vi "Tags.vi"(8 "error in (no error)":errorcluster, 11 "Node Ptr":T1 format="%.0x") -> (0 "error out":errorcluster)   [LabVIEW 2019, in "OPC UA Client Addon System Explorer.lvlib"]
uses:
  OPC UA Client Addon System Explorer.lvlib
  <vilib>/NI VeriStand/Custom Device API/Custom Device API.lvlib
  <vilib>/NI VeriStand/Custom Device API/Custom Device Item Ref.ctl
panel:
  in  "SHDocVw.IWebBrowser":refnum<k7>(container)
types:
  T1 = typedef "Custom Device API.lvlib/Custom Device Item Ref.ctl" = u64
  T2 = typedef "Custom Device API.lvlib/Custom Device Commands.ctl" = enum16{"Default", "Item renamed", "Shutdown", "Dynamic button pressed"}
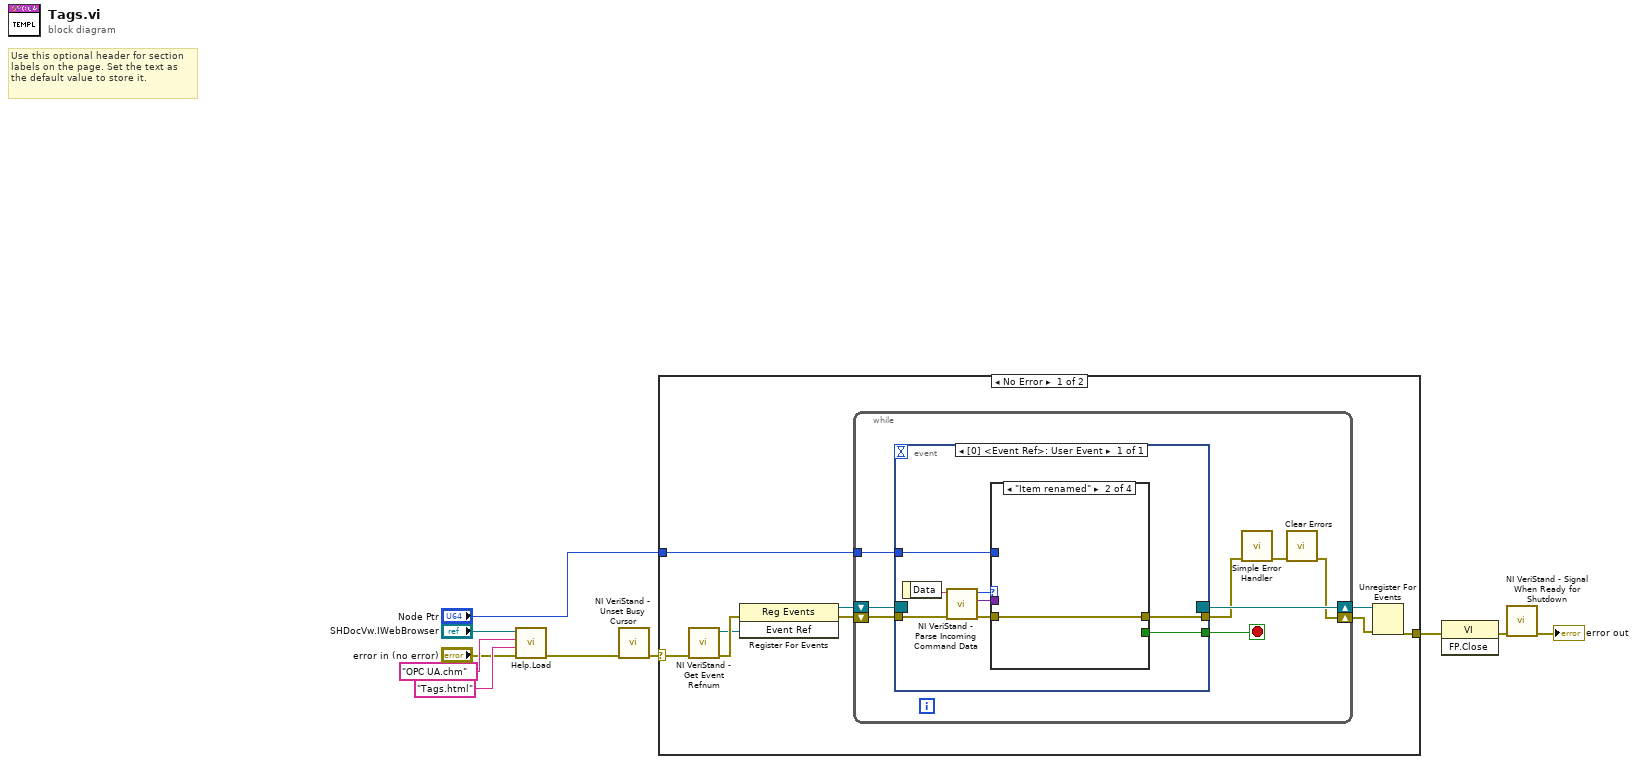
[diagram p0: block diagram]
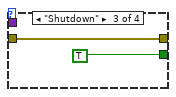
[diagram p3: hidden frame]
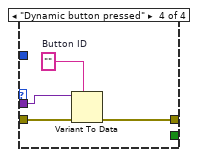
[diagram p4: hidden frame]
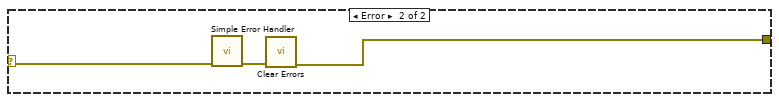
[diagram p5: hidden frame]
diagram:
  # "Use this optional header for section labels on the page. Set the text as the default value to store it."
  n1 = call "Help.Load.vi"("error in (no error)"="error in (no error)", "HTML File"="Tags.html" ("Main CHM File"), "Main CHM File"="OPC UA.chm", "SHDocVw.IWebBrowser2"="SHDocVw.IWebBrowser") -> ("error out"=w2:errorcluster)  [unwired: 7 in]
  n2 = call <vilib>:"NI VeriStand - Unset Busy Cursor.vi"("error in (no error)"=w2) -> ("error out"=w7:errorcluster)  [unwired: 10 out]
  n3 = case shown="No Error" w7 {
    selector: w7 -> [w11 w46]
    tunnel: [w16 w44] -> w10
    tunnel: "Node Ptr" -> [w12 _]
    frame No Error {
      n4 = call <vilib>:"NI VeriStand - Get Event Refnum.vi"("error in (no error)"=w11) -> ("error out"=w19:errorcluster, "Event Ref"=w15:refnum<user-event>)  [unwired: 9 out]
      n5 = register-events(error in=w19, w15) -> (reference out=w13:refnum<event-registration>, error out=w14:errorcluster)  [unwired: 1 in]
      n6 = while {
        tunnel: w12 -> [w23]
        shift-right: [w20] -> w17
        shift-left: w14 -> [w26]
        shift-right: [w27] -> w18
        shift-left: w13 -> [w25]
        stop <- w24 stop-if-true
        n7 = event shown="[0] <Event Ref>: User Event" {
          selector: w25 -> [_]
          dyn-events: [_] -> w27
          timeout: _ -> [_]
          tunnel: w26 -> [w35]
          tunnel: [w31] -> w24
          tunnel: [w30] -> w22
          tunnel: w23 -> [w29]
          event User Event {
            n8 = event-data() -> ("Data"=w34:string)  [unwired: 1 out]
            n9 = call <vilib>:"NI VeriStand - Parse Incoming Command Data.vi"("error in (no error)"=w35, "Incoming data"=w34) -> ("error out"=w33:errorcluster, "Outgoing data"=w28:variant, "Action"=w32:T2)  [unwired: 7 out]
            n10 = case shown="\"Item renamed\"" w32 {
              tunnel: w33 -> [w36 w37 w38 w43]
              tunnel: [_ _ TRUE _] -> w31
              tunnel: [w36 w37 w38 w40] -> w30
              tunnel: w29 -> [_ _ _ _]
              tunnel: w28 -> [_ _ _ w42]
              frame "Default", Default {
              }
              frame "Item renamed" {
              }
              frame "Shutdown" {
              }
              frame "Dynamic button pressed" {
                w41 = ""  # Button ID
                n11 = Variant To Data(error in=w43, type=w41, Variant=w42) -> (error out=w40:errorcluster)  [unwired: 1 out]
              }
            }
          }
        }
        n12 = call <vilib>:"Simple Error Handler.vi"("error in (no error)"=w22) -> ("error out"=w21:errorcluster)  [unwired: 1 in, 7 out]
        n13 = call <vilib>:"Clear Errors.vi"("error in (no error)"=w21) -> ("error out"=w20:errorcluster)  [unwired: 1 in, 5 out]
      }
      n14 = Unregister For Events(event registration refnum=w18, error in=w17) -> (error out=w16:errorcluster)
    }
    frame Error {
      n15 = call <vilib>:"Simple Error Handler.vi"("error in (no error)"=w46) -> ("error out"=w45:errorcluster)  [unwired: 1 in, 7 out]
      n16 = call <vilib>:"Clear Errors.vi"("error in (no error)"=w45) -> ("error out"=w44:errorcluster)  [unwired: 1 in, 5 out]
    }
  }
  n17 = invoke class="VI" method="FP.Close"(error in=w10) -> (error out=w9:errorcluster)  [unwired: 2 in, 2 out]
  n18 = call <vilib>:"NI VeriStand - Signal When Ready for Shutdown.vi"("error in (no error)"=w9) -> ("error out"=→"error out":errorcluster)  [unwired: 10 out]
